vi "Eye Movement Analyser.vi"(7 "Data Output":T12) -> ()   [LabVIEW 2016] (continued)
                      w89 = T14[] [enum."Check Save Status", enum."Chair"] items=["--- System ---", "Panel Monitoring", "Check Save Status", "Initialize", "Initialise GUI", "Quit", "--- Import ---", "Desaccade Time Data", "Desaccade Time Data Background", "Paint Delete", "Load Batch Log File", "Make Batch List", "Update Batch List", "Delete Batch List", "Delete Temporary LVS", "Save Temporary LVS", "Check for Batch LVS", "Process 3D Chinchilla", "Find default parameter", "Mars3D old", "Chair", "EyeSeeCam", "Open last session", "Save RAW", "Auto Impulse Parameter", "Save Image", "Wireless", "Process Coils Data", "Process JHOC Data", "Process Animal Data", "Australian Data", "ASCII", "Mars 3D", "Mars 3D Training", "Position Mean Plugin", "plot generator plugin", "Human VOG system", "Optotrak", "spline", "COR", "galvanic", "Generate New Time Plot", "Make off and gains permanent", "Generate New Impulse Plot", "Defer Impulse Plot", "Fill Impulse Plot Data", "Scale Impulse Plot", "Un-Defer Impulse Plot", "Snap Impulse Cursor", "Extract Saccades", "Impulse Analyser", "NTA", "Acceleration", "Saccade Velocity", "Horizontal Align", "Vertical Align", "Delete Impulse", "Cut Before", "Cut After", "Filter Data", "Undo Last", "Redo", "Mean and STD", "Group Analyser", "Generate Report", "Phase Plots", "Gain and Phase", "Example Plugin", "Time Constant Plugin", "Export Data", "Export Time Series Data", "Append Data", "Save Data", "Load Data", "Cut in Range", "Keep in range", "Stop"] ("State Stack (out)")
                    }
                    frame "txt", Default {
                      w91 = T14[] [] items=["--- System ---", "Panel Monitoring", "Check Save Status", "Initialize", "Initialise GUI", "Quit", "--- Import ---", "Desaccade Time Data", "Desaccade Time Data Background", "Paint Delete", "Load Batch Log File", "Make Batch List", "Update Batch List", "Delete Batch List", "Delete Temporary LVS", "Save Temporary LVS", "Check for Batch LVS", "Process 3D Chinchilla", "Find default parameter", "Mars3D old", "Chair", "EyeSeeCam", "Open last session", "Save RAW", "Auto Impulse Parameter", "Save Image", "Wireless", "Process Coils Data", "Process JHOC Data", "Process Animal Data", "Australian Data", "ASCII", "Mars 3D", "Mars 3D Training", "Position Mean Plugin", "plot generator plugin", "Human VOG system", "Optotrak", "spline", "COR", "galvanic", "Generate New Time Plot", "Make off and gains permanent", "Generate New Impulse Plot", "Defer Impulse Plot", "Fill Impulse Plot Data", "Scale Impulse Plot", "Un-Defer Impulse Plot", "Snap Impulse Cursor", "Extract Saccades", "Impulse Analyser", "NTA", "Acceleration", "Saccade Velocity", "Horizontal Align", "Vertical Align", "Delete Impulse", "Cut Before", "Cut After", "Filter Data", "Undo Last", "Redo", "Mean and STD", "Group Analyser", "Generate Report", "Phase Plots", "Gain and Phase", "Example Plugin", "Time Constant Plugin", "Export Data", "Export Time Series Data", "Append Data", "Save Data", "Load Data", "Cut in Range", "Keep in range", "Stop"] ("State Stack (out)")
                      n45 = One Button Dialog(message="File not handled") -> ()  [unwired: 1 in, 1 out]
                    }
                    frame "mars" {
                      w92 = T14[] [enum."Check Save Status", enum."Mars 3D"] items=["--- System ---", "Panel Monitoring", "Check Save Status", "Initialize", "Initialise GUI", "Quit", "--- Import ---", "Desaccade Time Data", "Desaccade Time Data Background", "Paint Delete", "Load Batch Log File", "Make Batch List", "Update Batch List", "Delete Batch List", "Delete Temporary LVS", "Save Temporary LVS", "Check for Batch LVS", "Process 3D Chinchilla", "Find default parameter", "Mars3D old", "Chair", "EyeSeeCam", "Open last session", "Save RAW", "Auto Impulse Parameter", "Save Image", "Wireless", "Process Coils Data", "Process JHOC Data", "Process Animal Data", "Australian Data", "ASCII", "Mars 3D", "Mars 3D Training", "Position Mean Plugin", "plot generator plugin", "Human VOG system", "Optotrak", "spline", "COR", "galvanic", "Generate New Time Plot", "Make off and gains permanent", "Generate New Impulse Plot", "Defer Impulse Plot", "Fill Impulse Plot Data", "Scale Impulse Plot", "Un-Defer Impulse Plot", "Snap Impulse Cursor", "Extract Saccades", "Impulse Analyser", "NTA", "Acceleration", "Saccade Velocity", "Horizontal Align", "Vertical Align", "Delete Impulse", "Cut Before", "Cut After", "Filter Data", "Undo Last", "Redo", "Mean and STD", "Group Analyser", "Generate Report", "Phase Plots", "Gain and Phase", "Example Plugin", "Time Constant Plugin", "Export Data", "Export Time Series Data", "Append Data", "Save Data", "Load Data", "Cut in Range", "Keep in range", "Stop"] ("State Stack (out)")
                    }
                    frame "lvs" {
                      w93 = T14[] [enum."Check Save Status", enum."Load Data"] items=["--- System ---", "Panel Monitoring", "Check Save Status", "Initialize", "Initialise GUI", "Quit", "--- Import ---", "Desaccade Time Data", "Desaccade Time Data Background", "Paint Delete", "Load Batch Log File", "Make Batch List", "Update Batch List", "Delete Batch List", "Delete Temporary LVS", "Save Temporary LVS", "Check for Batch LVS", "Process 3D Chinchilla", "Find default parameter", "Mars3D old", "Chair", "EyeSeeCam", "Open last session", "Save RAW", "Auto Impulse Parameter", "Save Image", "Wireless", "Process Coils Data", "Process JHOC Data", "Process Animal Data", "Australian Data", "ASCII", "Mars 3D", "Mars 3D Training", "Position Mean Plugin", "plot generator plugin", "Human VOG system", "Optotrak", "spline", "COR", "galvanic", "Generate New Time Plot", "Make off and gains permanent", "Generate New Impulse Plot", "Defer Impulse Plot", "Fill Impulse Plot Data", "Scale Impulse Plot", "Un-Defer Impulse Plot", "Snap Impulse Cursor", "Extract Saccades", "Impulse Analyser", "NTA", "Acceleration", "Saccade Velocity", "Horizontal Align", "Vertical Align", "Delete Impulse", "Cut Before", "Cut After", "Filter Data", "Undo Last", "Redo", "Mean and STD", "Group Analyser", "Generate Report", "Phase Plots", "Gain and Phase", "Example Plugin", "Time Constant Plugin", "Export Data", "Export Time Series Data", "Append Data", "Save Data", "Load Data", "Cut in Range", "Keep in range", "Stop"] ("State Stack (out)")
                    }
                  }
                  n46 = Bundle By Name(cluster=w86, "DC file"=w84) -> (w87:T17)
                }
                event "Batch Next": Mouse Down {
                  w98 = T14[] [enum."Save Temporary LVS", enum."Check for Batch LVS"] items=["--- System ---", "Panel Monitoring", "Check Save Status", "Initialize", "Initialise GUI", "Quit", "--- Import ---", "Desaccade Time Data", "Desaccade Time Data Background", "Paint Delete", "Load Batch Log File", "Make Batch List", "Update Batch List", "Delete Batch List", "Delete Temporary LVS", "Save Temporary LVS", "Check for Batch LVS", "Process 3D Chinchilla", "Find default parameter", "Mars3D old", "Chair", "EyeSeeCam", "Open last session", "Save RAW", "Auto Impulse Parameter", "Save Image", "Wireless", "Process Coils Data", "Process JHOC Data", "Process Animal Data", "Australian Data", "ASCII", "Mars 3D", "Mars 3D Training", "Position Mean Plugin", "plot generator plugin", "Human VOG system", "Optotrak", "spline", "COR", "galvanic", "Generate New Time Plot", "Make off and gains permanent", "Generate New Impulse Plot", "Defer Impulse Plot", "Fill Impulse Plot Data", "Scale Impulse Plot", "Un-Defer Impulse Plot", "Snap Impulse Cursor", "Extract Saccades", "Impulse Analyser", "NTA", "Acceleration", "Saccade Velocity", "Horizontal Align", "Vertical Align", "Delete Impulse", "Cut Before", "Cut After", "Filter Data", "Undo Last", "Redo", "Mean and STD", "Group Analyser", "Generate Report", "Phase Plots", "Gain and Phase", "Example Plugin", "Time Constant Plugin", "Export Data", "Export Time Series Data", "Append Data", "Save Data", "Load Data", "Cut in Range", "Keep in range", "Stop"] ("State Stack (out)")
                  n47 = event-data() -> ()  [unwired: 1 in, 7 out]
                  n48 = property on="Experiment Files" class="MCListbox (strict)"() -> ("Value"=w97:i32)  [unwired: 2 in, 2 out]
                  n49 = Increment(x=w97) -> (x+1=w96:i32)
                  n50 = property on="Experiment Files" class="MCListbox (strict)"("Value"=w96) -> ()  [unwired: 2 in, 2 out]
                }
                event "Load Batch File": Mouse Up {
                  w99 = T14[] [enum."Load Batch Log File"] items=["--- System ---", "Panel Monitoring", "Check Save Status", "Initialize", "Initialise GUI", "Quit", "--- Import ---", "Desaccade Time Data", "Desaccade Time Data Background", "Paint Delete", "Load Batch Log File", "Make Batch List", "Update Batch List", "Delete Batch List", "Delete Temporary LVS", "Save Temporary LVS", "Check for Batch LVS", "Process 3D Chinchilla", "Find default parameter", "Mars3D old", "Chair", "EyeSeeCam", "Open last session", "Save RAW", "Auto Impulse Parameter", "Save Image", "Wireless", "Process Coils Data", "Process JHOC Data", "Process Animal Data", "Australian Data", "ASCII", "Mars 3D", "Mars 3D Training", "Position Mean Plugin", "plot generator plugin", "Human VOG system", "Optotrak", "spline", "COR", "galvanic", "Generate New Time Plot", "Make off and gains permanent", "Generate New Impulse Plot", "Defer Impulse Plot", "Fill Impulse Plot Data", "Scale Impulse Plot", "Un-Defer Impulse Plot", "Snap Impulse Cursor", "Extract Saccades", "Impulse Analyser", "NTA", "Acceleration", "Saccade Velocity", "Horizontal Align", "Vertical Align", "Delete Impulse", "Cut Before", "Cut After", "Filter Data", "Undo Last", "Redo", "Mean and STD", "Group Analyser", "Generate Report", "Phase Plots", "Gain and Phase", "Example Plugin", "Time Constant Plugin", "Export Data", "Export Time Series Data", "Append Data", "Save Data", "Load Data", "Cut in Range", "Keep in range", "Stop"]  # State Stack (out)
                  n51 = event-data() -> ()  [unwired: 1 in, 7 out]
                }
                event "Btn Clear Temp LVS": Mouse Up {
                  w104 = T14[] [enum."Delete Batch List", enum."Delete Temporary LVS", enum."Make Batch List"] items=["--- System ---", "Panel Monitoring", "Check Save Status", "Initialize", "Initialise GUI", "Quit", "--- Import ---", "Desaccade Time Data", "Desaccade Time Data Background", "Paint Delete", "Load Batch Log File", "Make Batch List", "Update Batch List", "Delete Batch List", "Delete Temporary LVS", "Save Temporary LVS", "Check for Batch LVS", "Process 3D Chinchilla", "Find default parameter", "Mars3D old", "Chair", "EyeSeeCam", "Open last session", "Save RAW", "Auto Impulse Parameter", "Save Image", "Wireless", "Process Coils Data", "Process JHOC Data", "Process Animal Data", "Australian Data", "ASCII", "Mars 3D", "Mars 3D Training", "Position Mean Plugin", "plot generator plugin", "Human VOG system", "Optotrak", "spline", "COR", "galvanic", "Generate New Time Plot", "Make off and gains permanent", "Generate New Impulse Plot", "Defer Impulse Plot", "Fill Impulse Plot Data", "Scale Impulse Plot", "Un-Defer Impulse Plot", "Snap Impulse Cursor", "Extract Saccades", "Impulse Analyser", "NTA", "Acceleration", "Saccade Velocity", "Horizontal Align", "Vertical Align", "Delete Impulse", "Cut Before", "Cut After", "Filter Data", "Undo Last", "Redo", "Mean and STD", "Group Analyser", "Generate Report", "Phase Plots", "Gain and Phase", "Example Plugin", "Time Constant Plugin", "Export Data", "Export Time Series Data", "Append Data", "Save Data", "Load Data", "Cut in Range", "Keep in range", "Stop"] ("State Stack (out)")
                  n52 = event-data() -> ()  [unwired: 1 in, 8 out]
                }
                event "Update Batch File": Mouse Up {
                  w105 = T14[] [enum."Update Batch List"] items=["--- System ---", "Panel Monitoring", "Check Save Status", "Initialize", "Initialise GUI", "Quit", "--- Import ---", "Desaccade Time Data", "Desaccade Time Data Background", "Paint Delete", "Load Batch Log File", "Make Batch List", "Update Batch List", "Delete Batch List", "Delete Temporary LVS", "Save Temporary LVS", "Check for Batch LVS", "Process 3D Chinchilla", "Find default parameter", "Mars3D old", "Chair", "EyeSeeCam", "Open last session", "Save RAW", "Auto Impulse Parameter", "Save Image", "Wireless", "Process Coils Data", "Process JHOC Data", "Process Animal Data", "Australian Data", "ASCII", "Mars 3D", "Mars 3D Training", "Position Mean Plugin", "plot generator plugin", "Human VOG system", "Optotrak", "spline", "COR", "galvanic", "Generate New Time Plot", "Make off and gains permanent", "Generate New Impulse Plot", "Defer Impulse Plot", "Fill Impulse Plot Data", "Scale Impulse Plot", "Un-Defer Impulse Plot", "Snap Impulse Cursor", "Extract Saccades", "Impulse Analyser", "NTA", "Acceleration", "Saccade Velocity", "Horizontal Align", "Vertical Align", "Delete Impulse", "Cut Before", "Cut After", "Filter Data", "Undo Last", "Redo", "Mean and STD", "Group Analyser", "Generate Report", "Phase Plots", "Gain and Phase", "Example Plugin", "Time Constant Plugin", "Export Data", "Export Time Series Data", "Append Data", "Save Data", "Load Data", "Cut in Range", "Keep in range", "Stop"] ("State Stack (out)")
                  n53 = event-data() -> ()  [unwired: 1 in, 7 out]
                }
                event "Experiment Files": Value Change {
                  w110 = T14[] [enum."Save Temporary LVS", enum."Check for Batch LVS"] items=["--- System ---", "Panel Monitoring", "Check Save Status", "Initialize", "Initialise GUI", "Quit", "--- Import ---", "Desaccade Time Data", "Desaccade Time Data Background", "Paint Delete", "Load Batch Log File", "Make Batch List", "Update Batch List", "Delete Batch List", "Delete Temporary LVS", "Save Temporary LVS", "Check for Batch LVS", "Process 3D Chinchilla", "Find default parameter", "Mars3D old", "Chair", "EyeSeeCam", "Open last session", "Save RAW", "Auto Impulse Parameter", "Save Image", "Wireless", "Process Coils Data", "Process JHOC Data", "Process Animal Data", "Australian Data", "ASCII", "Mars 3D", "Mars 3D Training", "Position Mean Plugin", "plot generator plugin", "Human VOG system", "Optotrak", "spline", "COR", "galvanic", "Generate New Time Plot", "Make off and gains permanent", "Generate New Impulse Plot", "Defer Impulse Plot", "Fill Impulse Plot Data", "Scale Impulse Plot", "Un-Defer Impulse Plot", "Snap Impulse Cursor", "Extract Saccades", "Impulse Analyser", "NTA", "Acceleration", "Saccade Velocity", "Horizontal Align", "Vertical Align", "Delete Impulse", "Cut Before", "Cut After", "Filter Data", "Undo Last", "Redo", "Mean and STD", "Group Analyser", "Generate Report", "Phase Plots", "Gain and Phase", "Example Plugin", "Time Constant Plugin", "Export Data", "Export Time Series Data", "Append Data", "Save Data", "Load Data", "Cut in Range", "Keep in range", "Stop"] ("State Stack (out)")
                  n54 = event-data() -> ()  [unwired: 1 in, 5 out]
                }
                event "Impulse Trace": Mouse Move {
                  # "Is paint delete going to happen?"
                  # "Keep axis scaling to be restored after paint delete operation"
                  # "Cursor tool selected?"
                  n55 = event-data() -> ("Coords"=w128:T27)  [unwired: 1 in]
                  n56 = Unbundle By Name(w127) -> ("device ID"=w126:refnum<k1>)
                  n57 = call-poly <vilib>:"Acquire Input Data.vi"("device ID"=w126) -> ("button info"=w125:T28)  [unwired: 15 in, 3 out]
                  n58 = local read "Paint delete"() -> (w122:bool)
                  n59 = property on="Impulse Trace" class="WFGraph (strict)"() -> ("ActPaletteTool"=w124:i32)  [unwired: 2 in, 2 out]
                  n60 = Unbundle By Name(w125) -> ("button 1"=w111:bool)
                  n61 = local read "Fixed Amplitude"() -> (w119:bool)
                  n62 = local read "Fixed Time"() -> (w120:bool)
                  n63 = Equal To 0?(x=w124) -> (x = 0?=w123:bool)
                  n64 = Bundle("Fixed Time"=w120, "Fixed Amplitude"=w119) -> (w117:T29)  [unwired: 1 in]
                  n65 = Compound Arithmetic op=AND(w122, w111, w123) -> (w112:bool)
                  n66 = call <userlib>:"Boolean Trigger__ogtk.vi"("Boolean Input"=w112) -> ("Rising Edge"=w121:bool)  [unwired: 1 in, 1 out]
                  n67 = call-poly <userlib>:"Data Changed__ogtk.vi"("Boolean"=w112) -> ("Changed"=w116:bool)
                  n68 = call <userlib>:"Latch Value.vi"("Data in"=w117, "Set?"=w121) -> ("Data out"=w118:variant)
                  n69 = Variant To Data(type=w117, Variant=w118) -> (data=w115:T29)  [unwired: 1 in, 1 out]
                  n70 = Unbundle(w115) -> ("Fixed Time"=w114:bool, "Fixed Amplitude"=w113:bool)
                  n71 = case shown="True" w112 {
                    tunnel: [_ w140] -> w129
                    tunnel: w128 -> [_ w139]
                    frame False {
                      # "The user does not intend to delete impulses with the mouse. Do nothing."
                    }
                    frame True {
                      w140 = T14[] [enum."Paint Delete"] items=["--- System ---", "Panel Monitoring", "Check Save Status", "Initialize", "Initialise GUI", "Quit", "--- Import ---", "Desaccade Time Data", "Desaccade Time Data Background", "Paint Delete", "Load Batch Log File", "Make Batch List", "Update Batch List", "Delete Batch List", "Delete Temporary LVS", "Save Temporary LVS", "Check for Batch LVS", "Process 3D Chinchilla", "Find default parameter", "Mars3D old", "Chair", "EyeSeeCam", "Open last session", "Save RAW", "Auto Impulse Parameter", "Save Image", "Wireless", "Process Coils Data", "Process JHOC Data", "Process Animal Data", "Australian Data", "ASCII", "Mars 3D", "Mars 3D Training", "Position Mean Plugin", "plot generator plugin", "Human VOG system", "Optotrak", "spline", "COR", "galvanic", "Generate New Time Plot", "Make off and gains permanent", "Generate New Impulse Plot", "Defer Impulse Plot", "Fill Impulse Plot Data", "Scale Impulse Plot", "Un-Defer Impulse Plot", "Snap Impulse Cursor", "Extract Saccades", "Impulse Analyser", "NTA", "Acceleration", "Saccade Velocity", "Horizontal Align", "Vertical Align", "Delete Impulse", "Cut Before", "Cut After", "Filter Data", "Undo Last", "Redo", "Mean and STD", "Group Analyser", "Generate Report", "Phase Plots", "Gain and Phase", "Example Plugin", "Time Constant Plugin", "Export Data", "Export Time Series Data", "Append Data", "Save Data", "Load Data", "Cut in Range", "Keep in range", "Stop"] ("State Stack (out)")
                      # "The user intends to delete impulses with the mouse. Call paint delete and move the cursor to the mouse location."
                      n72 = invoke on="Impulse Trace" class="WFGraph (strict)" method="Map Coords To XY"("Coords"=w139) -> (error out=w137:errorcluster, "XY"=w138:cluster{"X":dbl, "Y":dbl})  [unwired: 6 in, 5 out]
                      n73 = property on="Impulse Trace" class="WFGraph (strict)"(error in=w137, "Cursor.Cursor Position"=w138) -> ()  [unwired: 1 in, 2 out]
                    }
                  }
                  n74 = case shown="True" w116 {
                    tunnel: w114 -> [_ w132]
                    tunnel: w113 -> [_ w131]
                    tunnel: w112 -> [_ w133]
                    frame False {
                    }
                    frame True {
                      # "Paint delete op started or stopped."
                      n75 = case shown="True" w133 {
                        tunnel: w132 -> [_ w136]
                        tunnel: w131 -> [_ w135]
                        frame True {
                          w134 = TRUE ("Fixed Time")
                          # "Started -> Fix Axes to prevent scaling during op."
                          n76 = local write "Fixed Time"(w134) -> ()
                          n77 = local write "Fixed Amplitude"(w134) -> ()
                        }
                        frame False {
                          # "Stopped -> Restore previous axis settings."
                          n78 = local write "Fixed Time"(w136) -> ()
                          n79 = local write "Fixed Amplitude"(w135) -> ()
                        }
                      }
                    }
                  }
                }
                event "Impulse Trace": Mouse Down? {
                  n80 = event-data() -> ("Button"=w143:u16)  [unwired: 1 in]
                  n81 = case shown="3" w143 {
                    frame Default {
                      # "Other button used. Do nothing."
                    }
                    frame 3 {
                      # "Panning tool"
                      # "Button 3 (middle) used. Set panning tool."
                      n82 = property on="Impulse Trace" class="WFGraph (strict)"("ActPaletteTool"=1 ("Palette:Active Tool")) -> ()  [unwired: 2 in, 2 out]
                    }
                  }
                  n83 = event-data() -> ()  [unwired: 2 in, 1 out]
                }
                event "Impulse Trace": Mouse Up {
                  n84 = event-data() -> ("Button"=w147:u16)  [unwired: 1 in]
                  n85 = case shown="3" w147 {
                    frame Default {
                      # "Other button used. Do nothing."
                    }
                    frame 3 {
                      # "selection cursor"
                      # "Button 3 (middle) used. Clear panning tool."
                      n86 = property on="Impulse Trace" class="WFGraph (strict)"("ActPaletteTool"=0 ("Palette:Active Tool")) -> ()  [unwired: 2 in, 2 out]
                    }
                  }
                }
                event Panel Close? {
                  w149 = T14[] [enum."Quit"] items=["--- System ---", "Panel Monitoring", "Check Save Status", "Initialize", "Initialise GUI", "Quit", "--- Import ---", "Desaccade Time Data", "Desaccade Time Data Background", "Paint Delete", "Load Batch Log File", "Make Batch List", "Update Batch List", "Delete Batch List", "Delete Temporary LVS", "Save Temporary LVS", "Check for Batch LVS", "Process 3D Chinchilla", "Find default parameter", "Mars3D old", "Chair", "EyeSeeCam", "Open last session", "Save RAW", "Auto Impulse Parameter", "Save Image", "Wireless", "Process Coils Data", "Process JHOC Data", "Process Animal Data", "Australian Data", "ASCII", "Mars 3D", "Mars 3D Training", "Position Mean Plugin", "plot generator plugin", "Human VOG system", "Optotrak", "spline", "COR", "galvanic", "Generate New Time Plot", "Make off and gains permanent", "Generate New Impulse Plot", "Defer Impulse Plot", "Fill Impulse Plot Data", "Scale Impulse Plot", "Un-Defer Impulse Plot", "Snap Impulse Cursor", "Extract Saccades", "Impulse Analyser", "NTA", "Acceleration", "Saccade Velocity", "Horizontal Align", "Vertical Align", "Delete Impulse", "Cut Before", "Cut After", "Filter Data", "Undo Last", "Redo", "Mean and STD", "Group Analyser", "Generate Report", "Phase Plots", "Gain and Phase", "Example Plugin", "Time Constant Plugin", "Export Data", "Export Time Series Data", "Append Data", "Save Data", "Load Data", "Cut in Range", "Keep in range", "Stop"]  # State Stack (out)
                  n87 = event-data() -> ()  [unwired: 1 in, 3 out]
                  n88 = event-data("Discard?"=TRUE) -> ()  [unwired: 1 in, 1 out]
                }
                event Value Change {
                  n89 = event-data() -> ("NewVal"=w155:T2)  [unwired: 1 in, 4 out]
                  n90 = Bundle By Name(cluster=w153, "Parameter Time Series"=w155) -> (w156:T30)
                }
                event Value Change {
                  n91 = event-data() -> ("NewVal"=w158:T8)  [unwired: 1 in, 4 out]
                  n92 = Bundle By Name(cluster=w160, "Parameter Impuls Series"=w158) -> (w159:T30)
                }
                event "Filter Method": Value Change {
                  w162 = T14[] [enum."Panel Monitoring"] items=["--- System ---", "Panel Monitoring", "Check Save Status", "Initialize", "Initialise GUI", "Quit", "--- Import ---", "Desaccade Time Data", "Desaccade Time Data Background", "Paint Delete", "Load Batch Log File", "Make Batch List", "Update Batch List", "Delete Batch List", "Delete Temporary LVS", "Save Temporary LVS", "Check for Batch LVS", "Process 3D Chinchilla", "Find default parameter", "Mars3D old", "Chair", "EyeSeeCam", "Open last session", "Save RAW", "Auto Impulse Parameter", "Save Image", "Wireless", "Process Coils Data", "Process JHOC Data", "Process Animal Data", "Australian Data", "ASCII", "Mars 3D", "Mars 3D Training", "Position Mean Plugin", "plot generator plugin", "Human VOG system", "Optotrak", "spline", "COR", "galvanic", "Generate New Time Plot", "Make off and gains permanent", "Generate New Impulse Plot", "Defer Impulse Plot", "Fill Impulse Plot Data", "Scale Impulse Plot", "Un-Defer Impulse Plot", "Snap Impulse Cursor", "Extract Saccades", "Impulse Analyser", "NTA", "Acceleration", "Saccade Velocity", "Horizontal Align", "Vertical Align", "Delete Impulse", "Cut Before", "Cut After", "Filter Data", "Undo Last", "Redo", "Mean and STD", "Group Analyser", "Generate Report", "Phase Plots", "Gain and Phase", "Example Plugin", "Time Constant Plugin", "Export Data", "Export Time Series Data", "Append Data", "Save Data", "Load Data", "Cut in Range", "Keep in range", "Stop"] ("State stack IN")
                  n93 = event-data() -> ("NewVal"=→"Tab Control 2":u16)  [unwired: 1 in, 4 out]
                }
                event "Time Curser Y1", "Time Curser X1", "Time Cursor Color 2", "Time Curser Y2", "Time Curser X2", "Time Cursor Color 1": Value Change {
                  n94 = event-data() -> ()  [unwired: 1 in, 5 out]
                  n95 = flat-sequence {
                    tunnel: [w177] -> w175
                    tunnel: [w177] -> w173
                    tunnel: [w176] -> w168
                    tunnel: w175 -> [w182]
                    tunnel: [w181] -> w174
                    tunnel: [w180] -> w169
                    frame #0 {
                      n96 = property on="Time Cursor Color 1" class="ColBox"() -> ("Value"=w178:u32)  [unwired: 2 in, 2 out]
                      n97 = property on="Time Curser X1" class="DigNum (strict)"() -> ("Value"=w177:dbl)  [unwired: 2 in, 2 out]
                      n98 = property on="Time Curser Y1" class="DigNum (strict)"() -> ("Value"=w176:dbl)  [unwired: 2 in, 2 out]
                      n99 = property on="Time series Trace" class="WFGraph (strict)"("Active Cursor"=u32 0, "Cursor.Cursor X"=w177, "Cursor.Cursor Y"=w176, "Cursor.Cursor Color"=w178) -> ()  [unwired: 2 in, 2 out]
                    }
                    frame #1 {
                      n100 = property on="Time Curser X2" class="DigNum (strict)"() -> ("Value"=w181:dbl)  [unwired: 2 in, 2 out]
                      n101 = property on="Time Cursor Color 2" class="ColBox"() -> ("Value"=w186:u32)  [unwired: 2 in, 2 out]
                      n102 = Less?(x=w181, y=w182) -> (x < y?=w184:bool)
                      n103 = case shown="True" w184 {
                        tunnel: [w187 w188] -> w183
                        tunnel: w181 -> [w187 _]
                        tunnel: w182 -> [_ w188]
                        frame False {
                        }
                        frame True {
                        }
                      }
                      n104 = property on="Time Curser Y2" class="DigNum (strict)"() -> ("Value"=w180:dbl)  [unwired: 2 in, 2 out]
                      n105 = property on="Time series Trace" class="WFGraph (strict)"("Active Cursor"=u32 1, "Cursor.Cursor X"=w183, "Cursor.Cursor Y"=w180, "Cursor.Cursor Color"=w186) -> ()  [unwired: 2 in, 2 out]
                    }
                  }
                  n106 = Subtract(x=w169, y=w168) -> (x-y=w167:dbl)
                  n107 = Subtract(x=w174, y=w173) -> (x-y=w172:dbl)
                  n108 = property on="dY" class="DigNum (strict)"("Value"=w167) -> ()  [unwired: 2 in, 2 out]
                  n109 = Multiply(x=w172, y=1000.0) -> (x*y=w170:dbl)
                  n110 = property on="dX" class="DigNum (strict)"("Value"=w170) -> ()  [unwired: 2 in, 2 out]
                }
                event "Time series Trace": Cursor Move {
                  n111 = event-data() -> ()  [unwired: 1 in, 8 out]
                  n112 = flat-sequence {
                    tunnel: [w205] -> w197
                    tunnel: [w204] -> w192
                    tunnel: [w208] -> w198
                    tunnel: [w207] -> w193
                    frame #0 {
                      n113 = property on="Time series Trace" class="WFGraph (strict)"("Active Cursor"=u32 0) -> ("Cursor.Cursor X"=w205:dbl, "Cursor.Cursor Y"=w204:dbl)  [unwired: 2 in, 2 out]
                      n114 = property on="Time Curser X1" class="DigNum (strict)"("Value"=w205) -> ()  [unwired: 2 in, 2 out]
                      n115 = property on="Time Curser Y1" class="DigNum (strict)"("Value"=w204) -> ()  [unwired: 2 in, 2 out]
                    }
                    frame #1 {
                      n116 = property on="Time series Trace" class="WFGraph (strict)"("Active Cursor"=u32 1) -> ("Cursor.Cursor X"=w208:dbl, "Cursor.Cursor Y"=w207:dbl)  [unwired: 2 in, 2 out]
                      n117 = property on="Time Curser Y2" class="DigNum (strict)"("Value"=w207) -> ()  [unwired: 2 in, 2 out]
                    }
                  }
                  n118 = Subtract(x=w198, y=w197) -> (x-y=w196:dbl)
                  n119 = Less?(x=w198, y=w197) -> (x < y?=w200:bool)
                  n120 = Subtract(x=w193, y=w192) -> (x-y=→"dY":dbl)
                  n121 = case shown="True" w200 {
                    tunnel: w197 -> [_ w202]
                    tunnel: [w201 w202] -> w199
                    tunnel: w198 -> [w201 _]
                    frame False {
                    }
                    frame True {
                      n122 = property on="Time series Trace" class="WFGraph (strict)"("Active Cursor"=u32 1, "Cursor.Cursor X"=w202) -> ()  [unwired: 2 in, 2 out]
                    }
                  }
                  n123 = Multiply(x=w196, y=1000.0) -> (x*y=→"dX":dbl)
                  n124 = property on="Time Curser X2" class="DigNum (strict)"("Value"=w199) -> ()  [unwired: 2 in, 2 out]
                }
                event "Auto Sort Parameter": Value Change {
                  w211 = T14[] [enum."Auto Impulse Parameter"] items=["--- System ---", "Panel Monitoring", "Check Save Status", "Initialize", "Initialise GUI", "Quit", "--- Import ---", "Desaccade Time Data", "Desaccade Time Data Background", "Paint Delete", "Load Batch Log File", "Make Batch List", "Update Batch List", "Delete Batch List", "Delete Temporary LVS", "Save Temporary LVS", "Check for Batch LVS", "Process 3D Chinchilla", "Find default parameter", "Mars3D old", "Chair", "EyeSeeCam", "Open last session", "Save RAW", "Auto Impulse Parameter", "Save Image", "Wireless", "Process Coils Data", "Process JHOC Data", "Process Animal Data", "Australian Data", "ASCII", "Mars 3D", "Mars 3D Training", "Position Mean Plugin", "plot generator plugin", "Human VOG system", "Optotrak", "spline", "COR", "galvanic", "Generate New Time Plot", "Make off and gains permanent", "Generate New Impulse Plot", "Defer Impulse Plot", "Fill Impulse Plot Data", "Scale Impulse Plot", "Un-Defer Impulse Plot", "Snap Impulse Cursor", "Extract Saccades", "Impulse Analyser", "NTA", "Acceleration", "Saccade Velocity", "Horizontal Align", "Vertical Align", "Delete Impulse", "Cut Before", "Cut After", "Filter Data", "Undo Last", "Redo", "Mean and STD", "Group Analyser", "Generate Report", "Phase Plots", "Gain and Phase", "Example Plugin", "Time Constant Plugin", "Export Data", "Export Time Series Data", "Append Data", "Save Data", "Load Data", "Cut in Range", "Keep in range", "Stop"] ("State Stack (out)")
                  n125 = event-data() -> ()  [unwired: 1 in, 5 out]
                }
                event "Accel Threshold [TH-1]", "Tolerance [ms]", "Impulse Plane 2", "Search Window [ms]", "Threshold 2 [% of TH-1]", "Only Use TH-2", "SD for Outlier detection", "Saccade width [ms]", "Velocity Threshold", "Impulse dir": Value Change {
                  n126 = event-data() -> ()  [unwired: 1 in, 5 out]
                  n127 = flat-sequence {
                    tunnel: w214 -> [w236]
                    tunnel: [w222] -> w217
                    tunnel: [w221] -> w216
                    tunnel: [w245] -> w219
                    tunnel: w217 -> [w243]
                    tunnel: w216 -> [w242]
                    tunnel: w214 -> [w241]
                    tunnel: [w240] -> w215
                    frame #0 {
                      n128 = disable-structure shown="Disabled" {
                        frame Disabled {
                          n129 = Wait (ms)(milliseconds to wait=u32 100) -> ()  [unwired: 1 out]
                        }
                        frame Enabled {
                        }
                      }
                    }
                    frame #1 {
                      n130 = local read "Accel Threshold [TH-1]"() -> (w234:dbl)
                      n131 = Unbundle By Name(w236) -> ("Data File.Sample Rate"=w237:i32, "desacc"=w235:T31)
                      n132 = local read "Impulse Plane 2"() -> (w239:T9)
                      n133 = local read "Tolerance [ms]"() -> (w233:dbl)
                      n134 = local read "Impulse dir"() -> (w238:bool)
                      n135 = Unbundle("Saccade width [ms]") -> (w231:i32, w230:i32)
                      n136 = Divide(x="Search Window [ms]", y=1000) -> (x/y=w224:dbl)
                      n137 = Bundle By Name(cluster=w235, "Threshold 2 [% of TH1]"="Threshold 2 [% of TH-1]", "Threshold 1 [Acc]"=w234, "tolerance"=w233, "Search WD"=w224, "always use TH2"="Only Use TH-2", "Range"="SD for Outlier detection", "Max time"=w231, "Min time"=w230, "Velocity Threshold"="Velocity Threshold") -> (w222:T31)
                      n138 = Bundle("Tolerance [ms]"=w233, "Accel Threshold [TH-1]"=w234, "Sample Rate"=w237, "Impulse Plane 2"=w239, "Impulse dir"=w238) -> (w221:T32)  [unwired: 1 in]
                    }
                    frame #2 {
                      n139 = case shown="True" "Live Update" {
                        tunnel: [_ w246] -> w245
                        frame False {
                        }
                        frame True {
                          w246 = T14[] [enum."Generate New Impulse Plot"] items=["--- System ---", "Panel Monitoring", "Check Save Status", "Initialize", "Initialise GUI", "Quit", "--- Import ---", "Desaccade Time Data", "Desaccade Time Data Background", "Paint Delete", "Load Batch Log File", "Make Batch List", "Update Batch List", "Delete Batch List", "Delete Temporary LVS", "Save Temporary LVS", "Check for Batch LVS", "Process 3D Chinchilla", "Find default parameter", "Mars3D old", "Chair", "EyeSeeCam", "Open last session", "Save RAW", "Auto Impulse Parameter", "Save Image", "Wireless", "Process Coils Data", "Process JHOC Data", "Process Animal Data", "Australian Data", "ASCII", "Mars 3D", "Mars 3D Training", "Position Mean Plugin", "plot generator plugin", "Human VOG system", "Optotrak", "spline", "COR", "galvanic", "Generate New Time Plot", "Make off and gains permanent", "Generate New Impulse Plot", "Defer Impulse Plot", "Fill Impulse Plot Data", "Scale Impulse Plot", "Un-Defer Impulse Plot", "Snap Impulse Cursor", "Extract Saccades", "Impulse Analyser", "NTA", "Acceleration", "Saccade Velocity", "Horizontal Align", "Vertical Align", "Delete Impulse", "Cut Before", "Cut After", "Filter Data", "Undo Last", "Redo", "Mean and STD", "Group Analyser", "Generate Report", "Phase Plots", "Gain and Phase", "Example Plugin", "Time Constant Plugin", "Export Data", "Export Time Series Data", "Append Data", "Save Data", "Load Data", "Cut in Range", "Keep in range", "Stop"] ("State Stack (out)")
                        }
                      }
                      n140 = Bundle By Name(cluster=w241, "desaccading parameters"=w242, "desacc"=w243) -> (w240:T30)
                    }
                  }
                  n141 = local write "Trace"(0 ("Trace")) -> ()
                }
                event "Impulse dir": Mouse Up {
                  w250 = T14[] [enum."Generate New Impulse Plot"] items=["--- System ---", "Panel Monitoring", "Check Save Status", "Initialize", "Initialise GUI", "Quit", "--- Import ---", "Desaccade Time Data", "Desaccade Time Data Background", "Paint Delete", "Load Batch Log File", "Make Batch List", "Update Batch List", "Delete Batch List", "Delete Temporary LVS", "Save Temporary LVS", "Check for Batch LVS", "Process 3D Chinchilla", "Find default parameter", "Mars3D old", "Chair", "EyeSeeCam", "Open last session", "Save RAW", "Auto Impulse Parameter", "Save Image", "Wireless", "Process Coils Data", "Process JHOC Data", "Process Animal Data", "Australian Data", "ASCII", "Mars 3D", "Mars 3D Training", "Position Mean Plugin", "plot generator plugin", "Human VOG system", "Optotrak", "spline", "COR", "galvanic", "Generate New Time Plot", "Make off and gains permanent", "Generate New Impulse Plot", "Defer Impulse Plot", "Fill Impulse Plot Data", "Scale Impulse Plot", "Un-Defer Impulse Plot", "Snap Impulse Cursor", "Extract Saccades", "Impulse Analyser", "NTA", "Acceleration", "Saccade Velocity", "Horizontal Align", "Vertical Align", "Delete Impulse", "Cut Before", "Cut After", "Filter Data", "Undo Last", "Redo", "Mean and STD", "Group Analyser", "Generate Report", "Phase Plots", "Gain and Phase", "Example Plugin", "Time Constant Plugin", "Export Data", "Export Time Series Data", "Append Data", "Save Data", "Load Data", "Cut in Range", "Keep in range", "Stop"] ("State Stack (out)")
                  n142 = event-data() -> ()  [unwired: 1 in, 7 out]
                  n143 = local write "Trace"(0 ("Trace")) -> ()
                }
                event "Reset to Raw": Value Change {
                  w251 = T14[] [enum."Generate New Time Plot", enum."Generate New Impulse Plot"] items=["--- System ---", "Panel Monitoring", "Check Save Status", "Initialize", "Initialise GUI", "Quit", "--- Import ---", "Desaccade Time Data", "Desaccade Time Data Background", "Paint Delete", "Load Batch Log File", "Make Batch List", "Update Batch List", "Delete Batch List", "Delete Temporary LVS", "Save Temporary LVS", "Check for Batch LVS", "Process 3D Chinchilla", "Find default parameter", "Mars3D old", "Chair", "EyeSeeCam", "Open last session", "Save RAW", "Auto Impulse Parameter", "Save Image", "Wireless", "Process Coils Data", "Process JHOC Data", "Process Animal Data", "Australian Data", "ASCII", "Mars 3D", "Mars 3D Training", "Position Mean Plugin", "plot generator plugin", "Human VOG system", "Optotrak", "spline", "COR", "galvanic", "Generate New Time Plot", "Make off and gains permanent", "Generate New Impulse Plot", "Defer Impulse Plot", "Fill Impulse Plot Data", "Scale Impulse Plot", "Un-Defer Impulse Plot", "Snap Impulse Cursor", "Extract Saccades", "Impulse Analyser", "NTA", "Acceleration", "Saccade Velocity", "Horizontal Align", "Vertical Align", "Delete Impulse", "Cut Before", "Cut After", "Filter Data", "Undo Last", "Redo", "Mean and STD", "Group Analyser", "Generate Report", "Phase Plots", "Gain and Phase", "Example Plugin", "Time Constant Plugin", "Export Data", "Export Time Series Data", "Append Data", "Save Data", "Load Data", "Cut in Range", "Keep in range", "Stop"] ("State stack IN")
                  n144 = event-data() -> ()  [unwired: 1 in, 5 out]
                }
                event "Reset Save Options": Mouse Down {
                  n145 = event-data() -> ()  [unwired: 1 in, 7 out]
                  n146 = Bundle By Name(cluster=w256, "Save Options"=FALSE) -> (w257:T17)
                }
                event "Display Saccade": Value Change {
                  w259 = T14[] [enum."Generate New Impulse Plot"] items=["--- System ---", "Panel Monitoring", "Check Save Status", "Initialize", "Initialise GUI", "Quit", "--- Import ---", "Desaccade Time Data", "Desaccade Time Data Background", "Paint Delete", "Load Batch Log File", "Make Batch List", "Update Batch List", "Delete Batch List", "Delete Temporary LVS", "Save Temporary LVS", "Check for Batch LVS", "Process 3D Chinchilla", "Find default parameter", "Mars3D old", "Chair", "EyeSeeCam", "Open last session", "Save RAW", "Auto Impulse Parameter", "Save Image", "Wireless", "Process Coils Data", "Process JHOC Data", "Process Animal Data", "Australian Data", "ASCII", "Mars 3D", "Mars 3D Training", "Position Mean Plugin", "plot generator plugin", "Human VOG system", "Optotrak", "spline", "COR", "galvanic", "Generate New Time Plot", "Make off and gains permanent", "Generate New Impulse Plot", "Defer Impulse Plot", "Fill Impulse Plot Data", "Scale Impulse Plot", "Un-Defer Impulse Plot", "Snap Impulse Cursor", "Extract Saccades", "Impulse Analyser", "NTA", "Acceleration", "Saccade Velocity", "Horizontal Align", "Vertical Align", "Delete Impulse", "Cut Before", "Cut After", "Filter Data", "Undo Last", "Redo", "Mean and STD", "Group Analyser", "Generate Report", "Phase Plots", "Gain and Phase", "Example Plugin", "Time Constant Plugin", "Export Data", "Export Time Series Data", "Append Data", "Save Data", "Load Data", "Cut in Range", "Keep in range", "Stop"] ("State Stack (out)")
                  n147 = event-data() -> ()  [unwired: 1 in, 5 out]
                }
                event "Paint delete": Value Change {
                  n148 = event-data() -> ("NewVal"=w266:bool)  [unwired: 1 in, 4 out]
                  n149 = Select(t=u32 0 ("Cursor.Cursor Mode"), s=w266, f=u32 1 ("Cursor.Cursor Mode")) -> (s? t:f=w263:u32)
                  n150 = property on="Impulse Trace" class="WFGraph (strict)"("Cursor.CursorMode"=w263) -> (error out=w267:errorcluster)  [unwired: 2 in, 1 out]
                  n151 = disable-structure shown="Disabled" {
                    disable-tunnel: [w271 _] -> w270
                    frame Disabled {
                      w271 = T14[] [enum."Paint Delete"] items=["--- System ---", "Panel Monitoring", "Check Save Status", "Initialize", "Initialise GUI", "Quit", "--- Import ---", "Desaccade Time Data", "Desaccade Time Data Background", "Paint Delete", "Load Batch Log File", "Make Batch List", "Update Batch List", "Delete Batch List", "Delete Temporary LVS", "Save Temporary LVS", "Check for Batch LVS", "Process 3D Chinchilla", "Find default parameter", "Mars3D old", "Chair", "EyeSeeCam", "Open last session", "Save RAW", "Auto Impulse Parameter", "Save Image", "Wireless", "Process Coils Data", "Process JHOC Data", "Process Animal Data", "Australian Data", "ASCII", "Mars 3D", "Mars 3D Training", "Position Mean Plugin", "plot generator plugin", "Human VOG system", "Optotrak", "spline", "COR", "galvanic", "Generate New Time Plot", "Make off and gains permanent", "Generate New Impulse Plot", "Defer Impulse Plot", "Fill Impulse Plot Data", "Scale Impulse Plot", "Un-Defer Impulse Plot", "Snap Impulse Cursor", "Extract Saccades", "Impulse Analyser", "NTA", "Acceleration", "Saccade Velocity", "Horizontal Align", "Vertical Align", "Delete Impulse", "Cut Before", "Cut After", "Filter Data", "Undo Last", "Redo", "Mean and STD", "Group Analyser", "Generate Report", "Phase Plots", "Gain and Phase", "Example Plugin", "Time Constant Plugin", "Export Data", "Export Time Series Data", "Append Data", "Save Data", "Load Data", "Cut in Range", "Keep in range", "Stop"] ("State Stack (out)")
                      # "This caused a bug where data would be deleted everytime the user swapped between paint delete/ no paint delete."
                    }
                    frame Enabled {
                    }
                  }
                  n152 = property on="Impulse Trace" class="WFGraph (strict)"(error in=w267) -> ("Cursor.Cursor X"=w262:dbl, "Cursor.Cursor Y"=w261:dbl)  [unwired: 1 in, 2 out]
                  n153 = local write "Impuls Cursor X"(w262) -> ()
                  n154 = local write "Impuls Cursor Y"(w261) -> ()
                }
                event "Impulse Trace": Cursor Move; "Delete Impulse": Key Up {
                  w272 = T14[] [enum."Snap Impulse Cursor", enum."Generate New Impulse Plot"] items=["--- System ---", "Panel Monitoring", "Check Save Status", "Initialize", "Initialise GUI", "Quit", "--- Import ---", "Desaccade Time Data", "Desaccade Time Data Background", "Paint Delete", "Load Batch Log File", "Make Batch List", "Update Batch List", "Delete Batch List", "Delete Temporary LVS", "Save Temporary LVS", "Check for Batch LVS", "Process 3D Chinchilla", "Find default parameter", "Mars3D old", "Chair", "EyeSeeCam", "Open last session", "Save RAW", "Auto Impulse Parameter", "Save Image", "Wireless", "Process Coils Data", "Process JHOC Data", "Process Animal Data", "Australian Data", "ASCII", "Mars 3D", "Mars 3D Training", "Position Mean Plugin", "plot generator plugin", "Human VOG system", "Optotrak", "spline", "COR", "galvanic", "Generate New Time Plot", "Make off and gains permanent", "Generate New Impulse Plot", "Defer Impulse Plot", "Fill Impulse Plot Data", "Scale Impulse Plot", "Un-Defer Impulse Plot", "Snap Impulse Cursor", "Extract Saccades", "Impulse Analyser", "NTA", "Acceleration", "Saccade Velocity", "Horizontal Align", "Vertical Align", "Delete Impulse", "Cut Before", "Cut After", "Filter Data", "Undo Last", "Redo", "Mean and STD", "Group Analyser", "Generate Report", "Phase Plots", "Gain and Phase", "Example Plugin", "Time Constant Plugin", "Export Data", "Export Time Series Data", "Append Data", "Save Data", "Load Data", "Cut in Range", "Keep in range", "Stop"] ("State Stack (out)")
                  n155 = event-data() -> ()  [unwired: 1 in, 3 out]
                  n156 = property on="Impulse Trace" class="WFGraph (strict)"() -> ("Cursor.Cursor X"=w276:dbl, "Cursor.Cursor Y"=w275:dbl)  [unwired: 2 in, 2 out]
                  n157 = property on="Impuls Cursor X" class="DigNum (strict)"("Value"=w276) -> ()  [unwired: 2 in, 2 out]
                  n158 = property on="Impuls Cursor Y" class="DigNum (strict)"("Value"=w275) -> ()  [unwired: 2 in, 2 out]
                }
                event "Impuls Cursor X", "Impuls Cursor Y": Value Change {
                  w277 = T14[] [enum."Snap Impulse Cursor", enum."Generate New Impulse Plot"] items=["--- System ---", "Panel Monitoring", "Check Save Status", "Initialize", "Initialise GUI", "Quit", "--- Import ---", "Desaccade Time Data", "Desaccade Time Data Background", "Paint Delete", "Load Batch Log File", "Make Batch List", "Update Batch List", "Delete Batch List", "Delete Temporary LVS", "Save Temporary LVS", "Check for Batch LVS", "Process 3D Chinchilla", "Find default parameter", "Mars3D old", "Chair", "EyeSeeCam", "Open last session", "Save RAW", "Auto Impulse Parameter", "Save Image", "Wireless", "Process Coils Data", "Process JHOC Data", "Process Animal Data", "Australian Data", "ASCII", "Mars 3D", "Mars 3D Training", "Position Mean Plugin", "plot generator plugin", "Human VOG system", "Optotrak", "spline", "COR", "galvanic", "Generate New Time Plot", "Make off and gains permanent", "Generate New Impulse Plot", "Defer Impulse Plot", "Fill Impulse Plot Data", "Scale Impulse Plot", "Un-Defer Impulse Plot", "Snap Impulse Cursor", "Extract Saccades", "Impulse Analyser", "NTA", "Acceleration", "Saccade Velocity", "Horizontal Align", "Vertical Align", "Delete Impulse", "Cut Before", "Cut After", "Filter Data", "Undo Last", "Redo", "Mean and STD", "Group Analyser", "Generate Report", "Phase Plots", "Gain and Phase", "Example Plugin", "Time Constant Plugin", "Export Data", "Export Time Series Data", "Append Data", "Save Data", "Load Data", "Cut in Range", "Keep in range", "Stop"] ("State Stack (out)")
                  # "THIS CASE MIGHT NEVER ACTUALLY BE CALLED?"
                  n159 = event-data() -> ()  [unwired: 1 in, 5 out]
                  n160 = property on="Impuls Cursor X" class="DigNum (strict)"() -> ("Value"=w278:dbl)  [unwired: 2 in, 2 out]
                  n161 = property on="Impuls Cursor Y" class="DigNum (strict)"() -> ("Value"=w279:dbl)  [unwired: 2 in, 2 out]
                  n162 = property on="Impulse Trace" class="WFGraph (strict)"("Cursor.Cursor X"=w278, "Cursor.Cursor Y"=w279) -> ()  [unwired: 2 in, 2 out]
                }
                event "Save Image Impulse": Mouse Down {
                  w283 = T14[] [enum."Save Image"] items=["--- System ---", "Panel Monitoring", "Check Save Status", "Initialize", "Initialise GUI", "Quit", "--- Import ---", "Desaccade Time Data", "Desaccade Time Data Background", "Paint Delete", "Load Batch Log File", "Make Batch List", "Update Batch List", "Delete Batch List", "Delete Temporary LVS", "Save Temporary LVS", "Check for Batch LVS", "Process 3D Chinchilla", "Find default parameter", "Mars3D old", "Chair", "EyeSeeCam", "Open last session", "Save RAW", "Auto Impulse Parameter", "Save Image", "Wireless", "Process Coils Data", "Process JHOC Data", "Process Animal Data", "Australian Data", "ASCII", "Mars 3D", "Mars 3D Training", "Position Mean Plugin", "plot generator plugin", "Human VOG system", "Optotrak", "spline", "COR", "galvanic", "Generate New Time Plot", "Make off and gains permanent", "Generate New Impulse Plot", "Defer Impulse Plot", "Fill Impulse Plot Data", "Scale Impulse Plot", "Un-Defer Impulse Plot", "Snap Impulse Cursor", "Extract Saccades", "Impulse Analyser", "NTA", "Acceleration", "Saccade Velocity", "Horizontal Align", "Vertical Align", "Delete Impulse", "Cut Before", "Cut After", "Filter Data", "Undo Last", "Redo", "Mean and STD", "Group Analyser", "Generate Report", "Phase Plots", "Gain and Phase", "Example Plugin", "Time Constant Plugin", "Export Data", "Export Time Series Data", "Append Data", "Save Data", "Load Data", "Cut in Range", "Keep in range", "Stop"] ("State Stack (out)")
                  n163 = event-data() -> ()  [unwired: 1 in, 7 out]
                }
                event "Reset To default": Mouse Down {
                  w288 = T14[] [enum."Generate New Impulse Plot"] items=["--- System ---", "Panel Monitoring", "Check Save Status", "Initialize", "Initialise GUI", "Quit", "--- Import ---", "Desaccade Time Data", "Desaccade Time Data Background", "Paint Delete", "Load Batch Log File", "Make Batch List", "Update Batch List", "Delete Batch List", "Delete Temporary LVS", "Save Temporary LVS", "Check for Batch LVS", "Process 3D Chinchilla", "Find default parameter", "Mars3D old", "Chair", "EyeSeeCam", "Open last session", "Save RAW", "Auto Impulse Parameter", "Save Image", "Wireless", "Process Coils Data", "Process JHOC Data", "Process Animal Data", "Australian Data", "ASCII", "Mars 3D", "Mars 3D Training", "Position Mean Plugin", "plot generator plugin", "Human VOG system", "Optotrak", "spline", "COR", "galvanic", "Generate New Time Plot", "Make off and gains permanent", "Generate New Impulse Plot", "Defer Impulse Plot", "Fill Impulse Plot Data", "Scale Impulse Plot", "Un-Defer Impulse Plot", "Snap Impulse Cursor", "Extract Saccades", "Impulse Analyser", "NTA", "Acceleration", "Saccade Velocity", "Horizontal Align", "Vertical Align", "Delete Impulse", "Cut Before", "Cut After", "Filter Data", "Undo Last", "Redo", "Mean and STD", "Group Analyser", "Generate Report", "Phase Plots", "Gain and Phase", "Example Plugin", "Time Constant Plugin", "Export Data", "Export Time Series Data", "Append Data", "Save Data", "Load Data", "Cut in Range", "Keep in range", "Stop"] ("State Stack (out)")
                  n164 = event-data() -> ()  [unwired: 1 in, 7 out]
                  n165 = call "Init Statemachine Data TD.vi"() -> ("output cluster"=w286:T30)  [unwired: 2 in]
                  n166 = Unbundle By Name(w286) -> ("desacc"=w285:T31)
                  n167 = Bundle By Name(cluster=w290, "desacc"=w285) -> (w289:T30)
                }
                event "Stop": Mouse Up {
                  w292 = T14[] [enum."Stop"] items=["--- System ---", "Panel Monitoring", "Check Save Status", "Initialize", "Initialise GUI", "Quit", "--- Import ---", "Desaccade Time Data", "Desaccade Time Data Background", "Paint Delete", "Load Batch Log File", "Make Batch List", "Update Batch List", "Delete Batch List", "Delete Temporary LVS", "Save Temporary LVS", "Check for Batch LVS", "Process 3D Chinchilla", "Find default parameter", "Mars3D old", "Chair", "EyeSeeCam", "Open last session", "Save RAW", "Auto Impulse Parameter", "Save Image", "Wireless", "Process Coils Data", "Process JHOC Data", "Process Animal Data", "Australian Data", "ASCII", "Mars 3D", "Mars 3D Training", "Position Mean Plugin", "plot generator plugin", "Human VOG system", "Optotrak", "spline", "COR", "galvanic", "Generate New Time Plot", "Make off and gains permanent", "Generate New Impulse Plot", "Defer Impulse Plot", "Fill Impulse Plot Data", "Scale Impulse Plot", "Un-Defer Impulse Plot", "Snap Impulse Cursor", "Extract Saccades", "Impulse Analyser", "NTA", "Acceleration", "Saccade Velocity", "Horizontal Align", "Vertical Align", "Delete Impulse", "Cut Before", "Cut After", "Filter Data", "Undo Last", "Redo", "Mean and STD", "Group Analyser", "Generate Report", "Phase Plots", "Gain and Phase", "Example Plugin", "Time Constant Plugin", "Export Data", "Export Time Series Data", "Append Data", "Save Data", "Load Data", "Cut in Range", "Keep in range", "Stop"] ("State Stack (out)")
                  n168 = event-data() -> ()  [unwired: 1 in, 7 out]
                }
                event "Process Coils Data": Mouse Up {
